vi "MoveRobot.vi"(0 "Error/Flow In":errorcluster, 1 "Reset":bool, 2 "Relative to Global Frame":bool, 7 "x (mm/s)":dbl(slide) scale=-1000.0..1000.0, 9 "y (mm/s)":dbl(slide) scale=-1000.0..1000.0, 11 "theta (rad/s)":dbl(slide) scale=-1.5..1.5, 12 "myRIO MXP Port A/B":tag="A/I2C", 13 "Controller ID#  (I2C Address)":u8=1 min=1 max=4, 14 "Controller ID#  (I2C Address) 2":u8=2 min=1 max=4) -> (4 "Error/Flow Out":errorcluster, 15 "Position":cluster{"X":dbl, "Y":dbl, "Theta":dbl})   [LabVIEW 2018]
uses:
  <vilib>/Analysis/coordinate.llb/2D Cartesian Coordinate Rotation (Scalar).vi
  <vilib>/imath/engines/lvmath2/RunTimeEngine/Managers/WorkSpace/UID Generator.vi
  <vilib>/imath/engines/lvmath2/RunTimeEngine/RangeToken/NIMS_Range_R2 - Integer.vi
  <instcachedir>/0/NIMS_Range_R2 - Integer_E35B921DECF84AADB7325A02D418BFCC.lvgen/NIMS_Range_R2 - Integer_E35B921DECF84AADB7325A02D418BFCC_000.vi
  <vilib>/imath/engines/lvmath2/RunTimeEngine/CommandStatement/MC_CommandStatement_break.vi
  <vilib>/imath/engines/lvmath2/RunTimeEngine/RunTimeType/NIMS_RunTimeType_From StrictType (excl LVString).vi
  <instcachedir>/0/NIMS_RunTimeType_From StrictType (excl LVString)_E7E34A65C99947108168652BAD14964D.lvgen/NIMS_RunTimeType_From StrictType (excl LVString)_E7E34A65C99947108168652BAD14964D_000.vi
  <vilib>/imath/engines/lvmath2/RunTimeEngine/LocalVariableDefStatement/MC_LocalVariableDefStatement_Display.vi
  <vilib>/imath/engines/lvmath2/RunTimeEngine/VariableToken/NIMS_VariableToken_CondDefinedDefinedByReplace.vi
  <instcachedir>/0/NIMS_VariableToken_CondDefinedDefinedByReplace_D162CFFC24174562A9FEA619A91E1A56.lvgen/NIMS_VariableToken_CondDefinedDefinedByReplace_D162CFFC24174562A9FEA619A91E1A56_002.vi
  <vilib>/imath/engines/lvmath2/RunTimeEngine/IndexReplace/NIMS V(S)=S.vi
  <instcachedir>/0/NIMS V(S)=S_420DA4522869420292A92FA3CC108C4E.lvgen/NIMS V(S)=S_420DA4522869420292A92FA3CC108C4E_000.vi
  <vilib>/imathl/engines/lvmath/Functions/Error Handling/Create Error.vi
  <vilib>/imath/engines/lvmath2/RunTimeEngine/VariableToken/NIMS_VariableToken_CondDefined.vi
  <instcachedir>/0/NIMS_VariableToken_CondDefined_BADDB804EBCA4B86883699DABD34B224.lvgen/NIMS_VariableToken_CondDefined_BADDB804EBCA4B86883699DABD34B224_003.vi
  <vilib>/imath/engines/lvmath2/RunTimeEngine/Managers/SymbolTable/Clear UID.vi
  <vilib>/imath/engines/lvmath2/RunTimeEngine/NodeEndStatement/NIMS_NodeEndStatement_Output.vi
  <instcachedir>/0/NIMS_NodeEndStatement_Output_53EC0D466D134D7ABD903AC30B43404B.lvgen/NIMS_NodeEndStatement_Output_53EC0D466D134D7ABD903AC30B43404B_005.vi
  <vilib>/imath/engines/lvmath2/RunTimeEngine/ErrorHandling/NIMS_Finalize Error.vi
  <vilib>/imath/engines/lvmath2/RunTimeEngine/IndexRead/NIMS V(S).vi
  <instcachedir>/0/NIMS V(S)_0488751826AF41519A22953C041130DC.lvgen/NIMS V(S)_0488751826AF41519A22953C041130DC_000.vi
  <vilib>/imath/engines/lvmath2/RunTimeEngine/ErrorHandling/NIMS_Create Error From Enums.vi
  <instcachedir>/0/NIMS_NodeEndStatement_Output_53EC0D466D134D7ABD903AC30B43404B.lvgen/NIMS_NodeEndStatement_Output_53EC0D466D134D7ABD903AC30B43404B_001.vi
  <vilib>/imath/engines/lvmath2/RunTimeEngine/Managers/SymbolTable/NIMS_WorkSpace.lvlib
  <vilib>/Analysis/NI_AALPro.lvlib
panel:
  in  "Wheel Radius":dbl=50.8
  in  "Robot Radius":dbl=149.0
  in  "Prev Encoders":i32[](array[numeric])
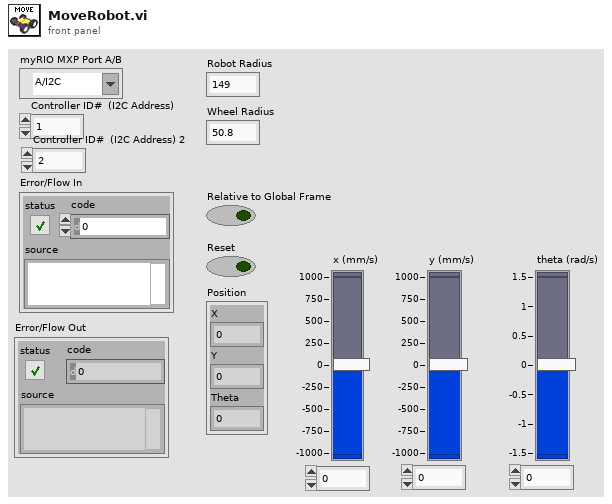
[diagram p1: front panel]
types:
  T1 = cluster{"x (mm/s)":dbl, "y (mm/s)":dbl, "theta (rad/s)":dbl}
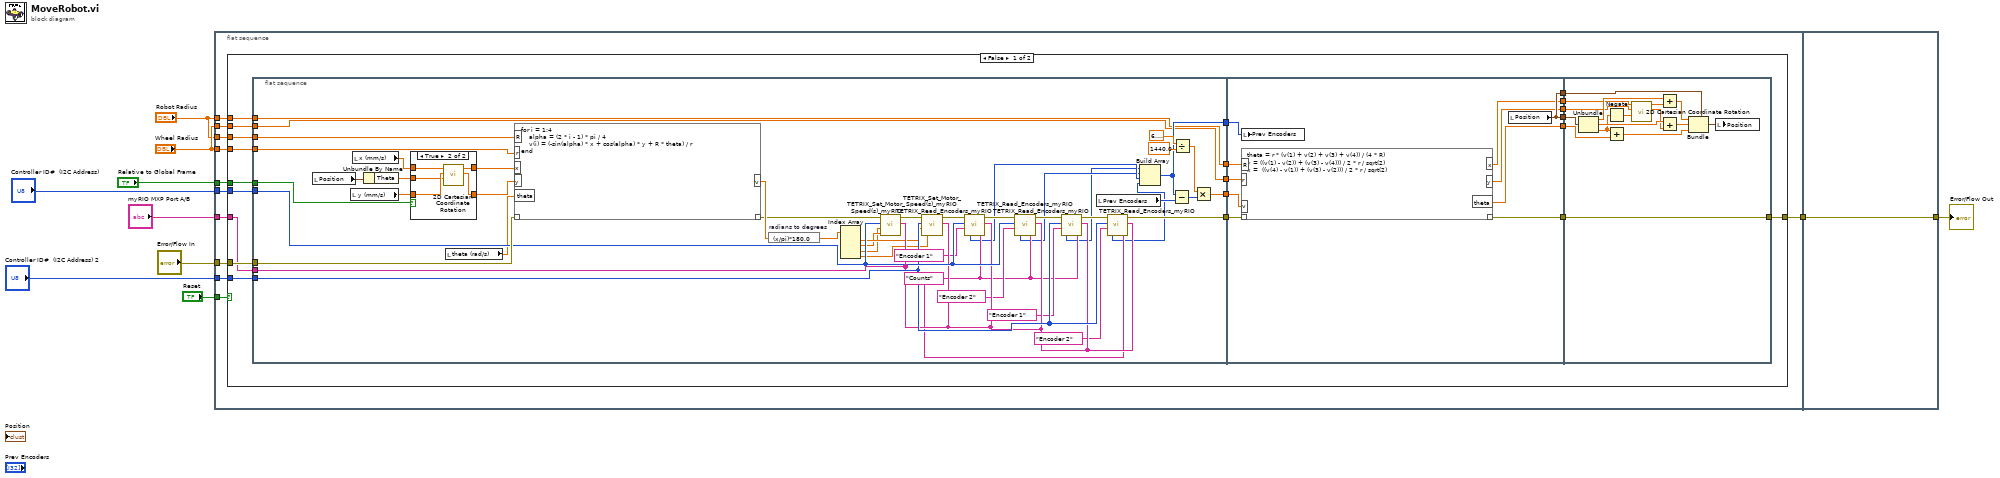
[diagram p0: block diagram]
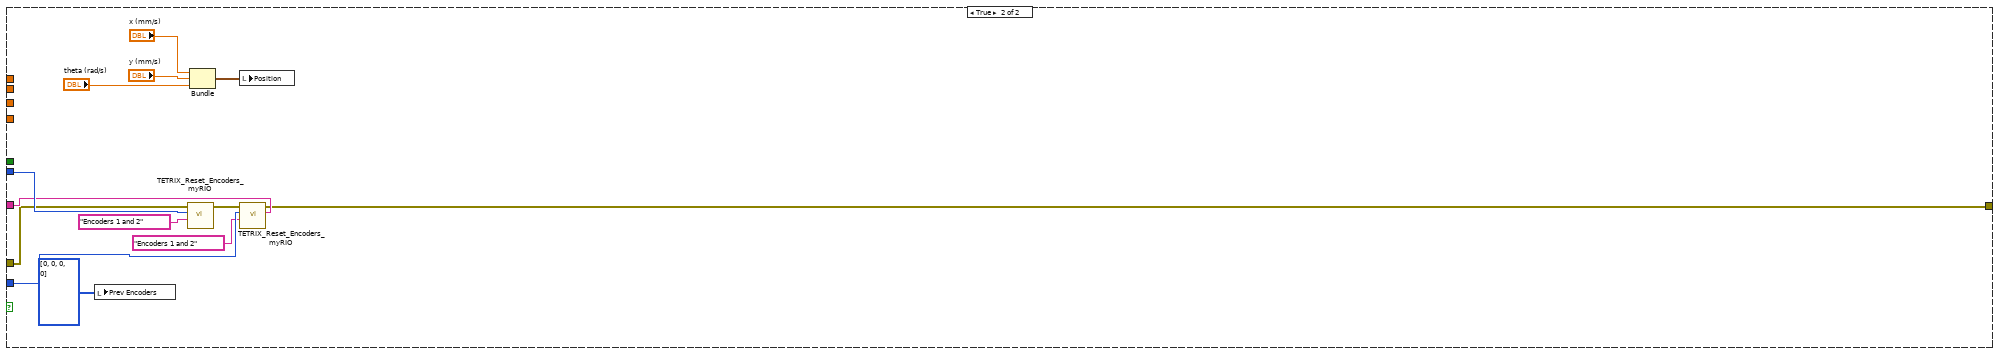
[diagram p3: hidden frame]
diagram:
  n1 = flat-sequence {
    tunnel: [w16] -> w9
    tunnel: "Reset" -> [w21]
    tunnel: "myRIO MXP Port A/B" -> [w20]
    tunnel: "Controller ID#  (I2C Address)" -> [w19]
    tunnel: "Controller ID#  (I2C Address) 2" -> [w18]
    tunnel: "Error/Flow In" -> [w17]
    tunnel: "Wheel Radius" -> [w15]
    tunnel: "Wheel Radius" -> [w14]
    tunnel: "Robot Radius" -> [w13]
    tunnel: "Robot Radius" -> [w12]
    tunnel: "Relative to Global Frame" -> [w11]
    tunnel: [w476] -> w10
    tunnel: w9 -> [w476]
    frame #0 {
      n2 = case shown="False" w21 {
        tunnel: w20 -> [w39 w466]
        tunnel: w19 -> [w41 w470]
        tunnel: w18 -> [w40 w467]
        tunnel: w17 -> [w42 w464]
        tunnel: [w32 w463] -> w16
        tunnel: w15 -> [w28 _]
        tunnel: w14 -> [w27 _]
        tunnel: w13 -> [w26 _]
        tunnel: w12 -> [w25 _]
        tunnel: w11 -> [w24 _]
        frame False {
          n3 = flat-sequence {
            tunnel: w42 -> [w87]
            tunnel: w41 -> [w79]
            tunnel: w40 -> [w78]
            tunnel: w39 -> [w76]
            tunnel: [w70] -> w38
            tunnel: [w64] -> w37
            tunnel: [w63] -> w36
            tunnel: [w60] -> w35
            tunnel: [w62] -> w34
            tunnel: w28 -> [w62]
            tunnel: w27 -> [w61]
            tunnel: w26 -> [w60]
            tunnel: w25 -> [w59]
            tunnel: w24 -> [w58]
            tunnel: w38 -> [w257]
            tunnel: w37 -> [w261]
            tunnel: w36 -> [w260]
            tunnel: w35 -> [w259]
            tunnel: w34 -> [w258]
            tunnel: [w256] -> w33
            tunnel: [w255] -> w31
            tunnel: [w255] -> w30
            tunnel: [w254] -> w29
            tunnel: [w253] -> w23
            tunnel: [w252] -> w22
            tunnel: w33 -> [w462]
            tunnel: w31 -> [w460]
            tunnel: w30 -> [w459]
            tunnel: w29 -> [w454]
            tunnel: [w462] -> w32
            tunnel: w23 -> [w452]
            tunnel: w22 -> [w450]
            frame #0 {
              w71 = "Counts" ("Encoder Units")
              n4 = local read "Position"() -> (w52:cluster{"X":dbl, "Y":dbl, "Theta":dbl})
              n5 = local read "y (mm/s)"() -> (w56:dbl)
              n6 = local read "x (mm/s)"() -> (w57:dbl)
              n7 = Unbundle By Name(w52) -> ("Theta"=w51:dbl)
              n8 = case shown="True" w58 {
                tunnel: w57 -> [w89 w94]
                tunnel: w56 -> [w88 w93]
                tunnel: [w89 w92] -> w55
                tunnel: [w88 w91] -> w54
                tunnel: w51 -> [_ w90]
                frame False {
                }
                frame True {
                  n9 = call-poly <vilib>:"2D Cartesian Coordinate Rotation.vi"("theta"=w90, "y"=w93, "x"=w94) -> ("y out"=w91:dbl, "x out"=w92:dbl)  [unwired: 6 in, 1 out]
                }
              }
              n10 = local read "theta (rad/s)"() -> (w53:dbl)
              n11 = mathscript code="for i = 1:4\n    alpha = (2 * i - 1) * pi / 4\n    v(i) = (-sin(alpha) * x + cos(alpha) * y + R * theta) / r\nend"("??"=w87, "R"=w59, "r"=w61, "x"=w55, "y"=w54, "theta"=w53) -> ("??"=w84:errorcluster, "v"=w86:dbl[])
              n12 = expression code="(x/pi)*180.0" "radians to degrees"(w86) -> (w85:dbl[])
              n13 = Index Array(array=w85) -> (element #1=w50:dbl, element #2=w49:dbl, element #3=w48:dbl, element #4=w47:dbl)  [unwired: 4 in]
              n14 = call <vilib>:"TETRIX_Set_Motor_Speed(s)_myRIO.vi"("myRIO MXP Port A/B"=w76, "Motor 2 Speed (Degrees per second). Sign (+/-)  sets direction."=w49, "Motor 1 Speed (Degrees per second). Sign (+/-)  sets direction."=w48, "Controller ID#  (I2C Address)"=w79, "Error/Flow In"=w84) -> ("Error/Flow Out"=w83:errorcluster)  [unwired: 2 in]
              n15 = call <vilib>:"TETRIX_Set_Motor_Speed(s)_myRIO.vi"("myRIO MXP Port A/B"=w76, "Motor 2 Speed (Degrees per second). Sign (+/-)  sets direction."=w47, "Motor 1 Speed (Degrees per second). Sign (+/-)  sets direction."=w50, "Controller ID#  (I2C Address)"=w78, "Error/Flow In"=w83) -> ("Error/Flow Out"=w82:errorcluster)  [unwired: 2 in]
              n16 = call <vilib>:"TETRIX_Read_Encoders_myRIO.vi"("Encoder Units"=w71, "myRIO MXP Port A/B"=w76, "Select Encoder"="Encoder 1", "Controller ID#  (I2C Address)"=w79, "Error/Flow In"=w82) -> ("Error/Flow Out"=w81:errorcluster, "Encoder Output"=w46:i32)  [unwired: 1 in]
              n17 = call <vilib>:"TETRIX_Read_Encoders_myRIO.vi"("Encoder Units"=w71, "myRIO MXP Port A/B"=w76, "Select Encoder"="Encoder 2", "Controller ID#  (I2C Address)"=w79, "Error/Flow In"=w81) -> ("Error/Flow Out"=w80:errorcluster, "Encoder Output"=w45:i32)  [unwired: 1 in]
              n18 = call <vilib>:"TETRIX_Read_Encoders_myRIO.vi"("Encoder Units"=w71, "myRIO MXP Port A/B"=w76, "Select Encoder"="Encoder 1", "Controller ID#  (I2C Address)"=w78, "Error/Flow In"=w80) -> ("Error/Flow Out"=w77:errorcluster, "Encoder Output"=w44:i32)  [unwired: 1 in]
              n19 = local read "Prev Encoders"() -> (w69:i32[])
              n20 = call <vilib>:"TETRIX_Read_Encoders_myRIO.vi"("Encoder Units"=w71, "myRIO MXP Port A/B"=w76, "Select Encoder"="Encoder 2", "Controller ID#  (I2C Address)"=w78, "Error/Flow In"=w77) -> ("Error/Flow Out"=w70:errorcluster, "Encoder Output"=w43:i32)  [unwired: 1 in]
              n21 = Build Array(w44, w45, w46, w43) -> (w64:i32[])
              n22 = Subtract(x=w64, y=w69) -> (x-y=w65:i32[])
              n23 = Divide(x=6.283185307179586, y=1440.0) -> (x/y=w68:dbl)
              n24 = Multiply(x=w68, y=w65) -> (x*y=w63:dbl[])
            }
            frame #1 {
              n25 = local write "Prev Encoders"(w261) -> ()
              n26 = mathscript code="theta = r * (v(1) + v(2) + v(3) + v(4)) / (4 * R)\ny = ((v(1) - v(2)) + (v(3) - v(4))) / 2 * r / sqrt(2)\nx =  ((v(4) - v(1)) + (v(3) - v(2))) / 2 * r / sqrt(2)"("??"=w257, "v"=w260, "r"=w258, "R"=w259) -> ("??"=w256:errorcluster, "x"=w253:dbl, "y"=w252:dbl, "theta"=w254:dbl)
              n27 = local read "Position"() -> (w255:cluster{"X":dbl, "Y":dbl, "Theta":dbl})
            }
            frame #2 {
              n28 = Unbundle(w459) -> ("X"=w458:dbl, "Y"=w456:dbl, "Theta"=w448:dbl)
              n29 = Negate(x=w448) -> (-x=w447:dbl)
              n30 = Add(x=w448, y=w454) -> (x+y=w453:dbl)
              n31 = call-poly <vilib>:"2D Cartesian Coordinate Rotation.vi"("theta"=w447, "y"=w450, "x"=w452) -> ("y out"=w449:dbl, "x out"=w451:dbl)  [unwired: 6 in, 1 out]
              n32 = Add(x=w458, y=w451) -> (x+y=w457:dbl)
              n33 = Add(x=w456, y=w449) -> (x+y=w455:dbl)
              n34 = Bundle(cluster=w460, "X"=w457, "Y"=w455, "Theta"=w453) -> (w461:cluster{"X":dbl, "Y":dbl, "Theta":dbl})
              n35 = local write "Position"(w461) -> ()
            }
          }
        }
        frame True {
          n36 = local write "Prev Encoders"(i32[] [0, 0, 0, 0] ("Prev Encoders")) -> ()
          n37 = call <vilib>:"TETRIX_Reset_Encoders_myRIO.vi"("Select Encoder"="Encoders 1 and 2", "Controller ID#  (I2C Address)"=w470, "Error/Flow In"=w464) -> ("Error/Flow Out"=w468:errorcluster)  [unwired: 4 in]
          n38 = Bundle("x (mm/s)"="x (mm/s)", "y (mm/s)"="y (mm/s)", "theta (rad/s)"="theta (rad/s)") -> (w472:T1)  [unwired: 1 in]
          n39 = local write "Position"(w472) -> ()
          n40 = call <vilib>:"TETRIX_Reset_Encoders_myRIO.vi"("myRIO MXP Port A/B"=w466, "Select Encoder"="Encoders 1 and 2", "Controller ID#  (I2C Address)"=w467, "Error/Flow In"=w468) -> ("Error/Flow Out"=w463:errorcluster)  [unwired: 3 in]
        }
      }
    }
    frame #1 {
    }
  }
  "Error/Flow Out" <- w10
